vi "Elliptic Integral of the 2nd kind.vi"   [LabVIEW 2014, in "NI_Gmath.lvlib"]
doc: "Computes the Legendre elliptic integral of the second kind. You must manually select the polymorphic instance you want to use."
uses:
  NI_Gmath.lvlib
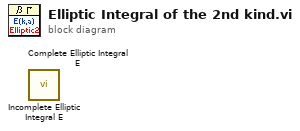
[diagram p0: block diagram]
diagram:
  n1 = call "Incomplete Elliptic Integral E.vi"() -> ()  [unwired: 11 in, 1 out]
  n2 = call "Complete Elliptic Integral E.vi"() -> ()  [unwired: 11 in, 1 out]
